vi "_MobileTest_Consume.vi"(9 "ID":u32) -> (2 "Data":variant)   [LabVIEW 2019]
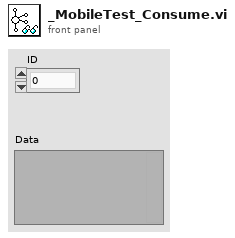
[diagram p1: front panel]
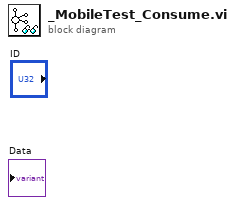
[diagram p0: block diagram]
diagram:
